vi "Capture Settings.vi"(0 "Notifier Name":string, 5 "Save Path":path, 9 "Num of Frames":u32, 11 "Error In":errorcluster) -> (4 "Notifier Name DUP":string, 15 "Error Out":errorcluster)   [LabVIEW 2020]
uses:
  Hardware Configuration/Hardware Configuration Controls/Company.ctl
  Hamamatsu/Orca Flash/Orca Flash Controls/Orca Flash Actions.ctl
  IDS/IDS Controls/IDS Actions.ctl
  Photometrics/Prime BSI/R Cubed SITK/Prime BSI R3 Controls/Prime R3 Actions.ctl
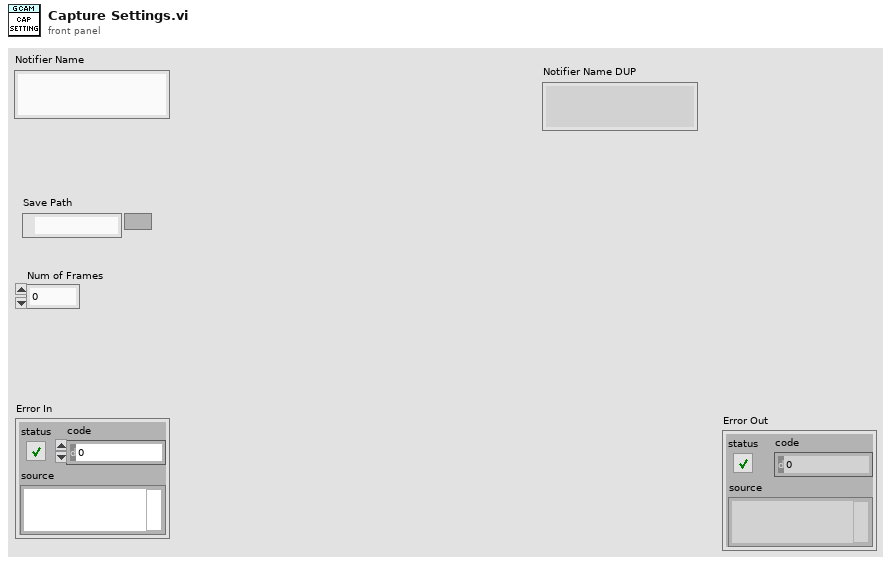
[diagram p1: front panel]
types:
  T1 = typedef "Company.ctl" = enum16{"AA Opto Electronic", "ASI", "Coherent", "Creset Optics", "CVI", "DAQmx", "Hamamatsu", "IDS", "Mad City Labs", "Marzhauser", "Measurement Computing", "MPB Com", "Olympus", "Photometrics", "PI", "Prior", "Thorlabs"}
  T2 = typedef "Orca Flash Actions.ctl" = enum16{"Idle", "Preview", "Record", "Record Settings", "Set Param", "Get Param", "Set ROI", "Get ROI", "Trigger Source", "Trigger Type", "Progessive Mode", "Area Mode", "Status", "Quit"}
  T3 = typedef "IDS Actions.ctl" = enum16{"Error Check", "Initialize", "Preview", "Record", "Abort", "Record Settings", "Set Parameter", "Get Parameter", "Set ROI", "Get ROI", "Status", "Quit"}
  T4 = typedef "Prime R3 Actions.ctl" = enum16{"Error Check", "Initialize", "Preview", "Record", "Abort", "Record Settings", "Set Parameter", "Get Parameter", "Set ROI", "Get ROI", "Status", "Set Trigger", "Quit"}
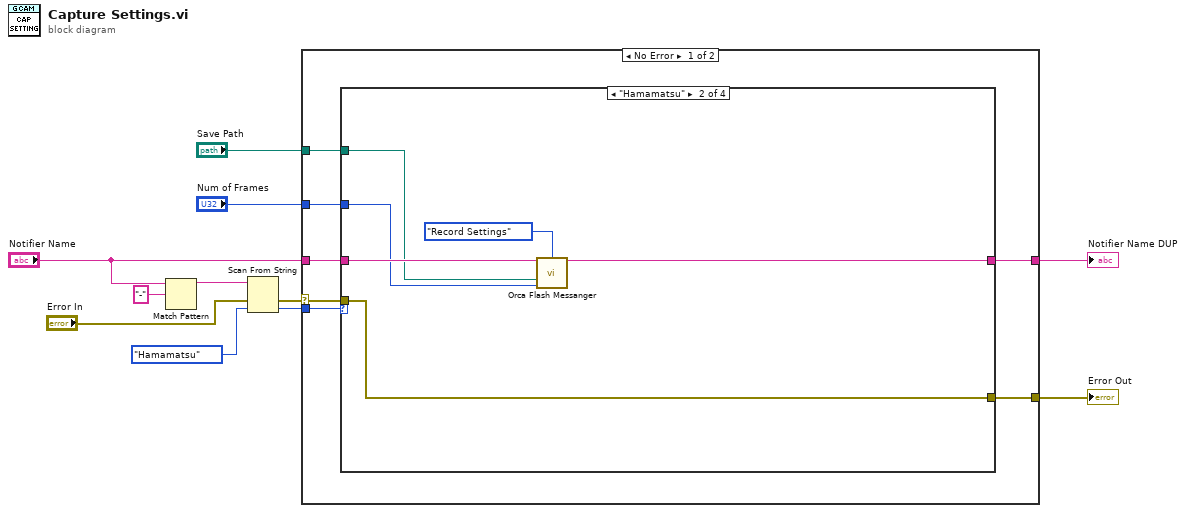
[diagram p0: block diagram]
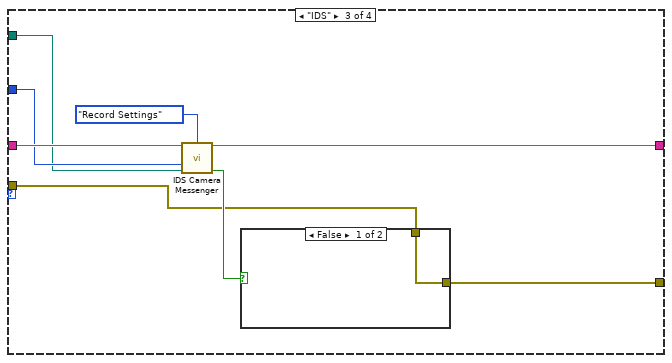
[diagram p3: hidden frame]
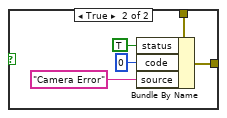
[diagram p4: hidden frame]
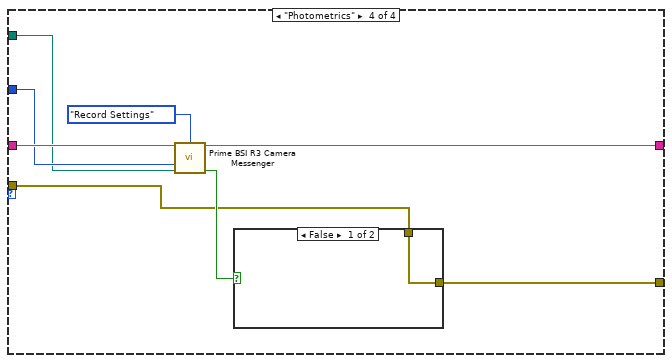
[diagram p5: hidden frame]
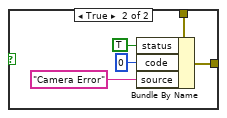
[diagram p6: hidden frame]
diagram:
  n1 = Match Pattern(string="Notifier Name", regular expression="-") -> (before substring=w9:string)  [unwired: 1 in, 3 out]
  n2 = Scan From String(input string=w9, error in="Error In", default 1=Company."Hamamatsu" ("Company")) -> (error out=w5:errorcluster, output 1=w8:T1)  [unwired: 2 in, 2 out]
  n3 = case shown="No Error" w5 {
    selector: w5 -> [w16 w55]
    tunnel: w8 -> [w18 _]
    tunnel: "Notifier Name" -> [w17 w56]
    tunnel: [w15 w56] -> w4
    tunnel: [w14 w55] -> w3
    tunnel: "Num of Frames" -> [w13 _]
    tunnel: "Save Path" -> [w12 _]
    frame No Error {
      n4 = case shown="\"Hamamatsu\"" w18 {
        tunnel: w17 -> [w20 w26 w34 w48]
        tunnel: w16 -> [w19 w23 w30 w45]
        tunnel: [w20 w24 w33 w47] -> w15
        tunnel: [w19 w23 w29 w44] -> w14
        tunnel: w13 -> [_ w22 w28 w42]
        tunnel: w12 -> [_ w21 w27 w41]
        frame Default {
        }
        frame "Hamamatsu" {
          n5 = call "Orca Flash Messanger.vi"("Notifier Name"=w26, "Camera Actions"=Orca_Flash_Actions."Record Settings", "Path"=w21, "# of frames"=w22) -> ("Notifier Name Dup"=w24:string)  [unwired: 7 in, 4 out]
        }
        frame "IDS" {
          n6 = call "IDS Camera Messenger.vi"("Notifier Name"=w34, "IDS Actions"=IDS_Actions."Record Settings", "# of Frames"=w28, "File Save Path"=w27) -> ("Notifier Name (Dup)"=w33:string, "Error?"=w31:bool)  [unwired: 6 in, 4 out]
          n7 = case shown="False" w31 {
            tunnel: w30 -> [w35 w40]
            tunnel: [w35 w39] -> w29
            frame False {
            }
            frame True {
              n8 = Bundle By Name(cluster=w40, "status"=TRUE, "code"=0, "source"="Camera Error") -> (w39:errorcluster)
            }
          }
        }
        frame "Photometrics" {
          n9 = call "Prime BSI R3 Camera Messenger.vi"("Notifier Name"=w48, "Prime Actions"=Prime_R3_Actions."Record Settings", "# of Frames"=w42, "File Save Path"=w41) -> ("Notifier Name (Dup)"=w47:string, "Error?"=w46:bool)  [unwired: 6 in, 4 out]
          n10 = case shown="False" w46 {
            tunnel: w45 -> [w49 w54]
            tunnel: [w49 w53] -> w44
            frame False {
            }
            frame True {
              n11 = Bundle By Name(cluster=w54, "status"=TRUE, "code"=0, "source"="Camera Error") -> (w53:errorcluster)
            }
          }
        }
      }
    }
    frame Error {
    }
  }
  "Error Out" <- w3
  "Notifier Name DUP" <- w4
